vi "SW_Fire_TTL_on_start_or_stop.vi"(7 "TTL pulse length, ms":dbl=250.0 format="%#_13g", 8 "error in (no error)":errorcluster, 9 "Serial Port In":refnum<visa-resource-name>="COM3", 10 "Flush receive buffer?":bool=TRUE, 11 "IO parameters cluster in":T1) -> (0 "error out":errorcluster, 1 "Serial Port Out":refnum<visa-resource-name>="COM3", 3 "Time spent to process command, s":dbl=250.0)   [LabVIEW 2018, in "Tracker.lvlib"]
doc: "Fires TTL High to the TTL2 output for ~250 ms (default)."
uses:
  Tracker.lvlib
  Controls/CTL_IO_params_cluster.ctl
  <vilib>/Instr/_visa.llb/VISA Flush IO Buffer Mask.ctl
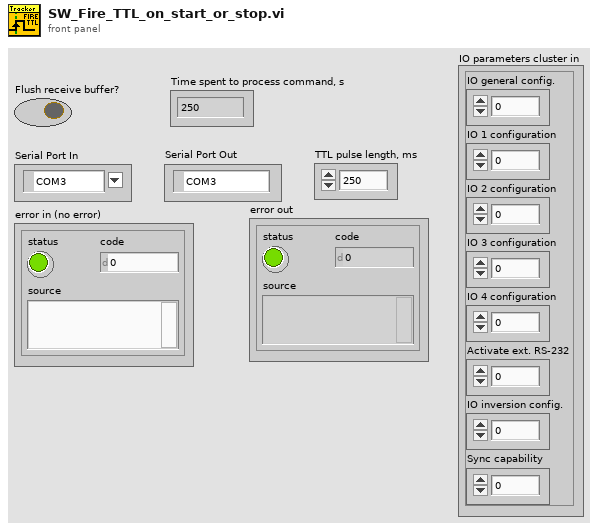
[diagram p1: front panel]
types:
  T1 = typedef "Tracker.lvlib/CTL_IO_params_cluster.ctl" = cluster{"IO general config.":u16, "IO 1 configuration":u16, "IO 2 configuration":u16, "IO 3 configuration":u16, "IO 4 configuration":u16, "Activate ext. RS-232":u16, "IO inversion config.":u16, "Sync capability":u8}
  T2 = typedef "VISA Flush IO Buffer Mask.ctl" = u16
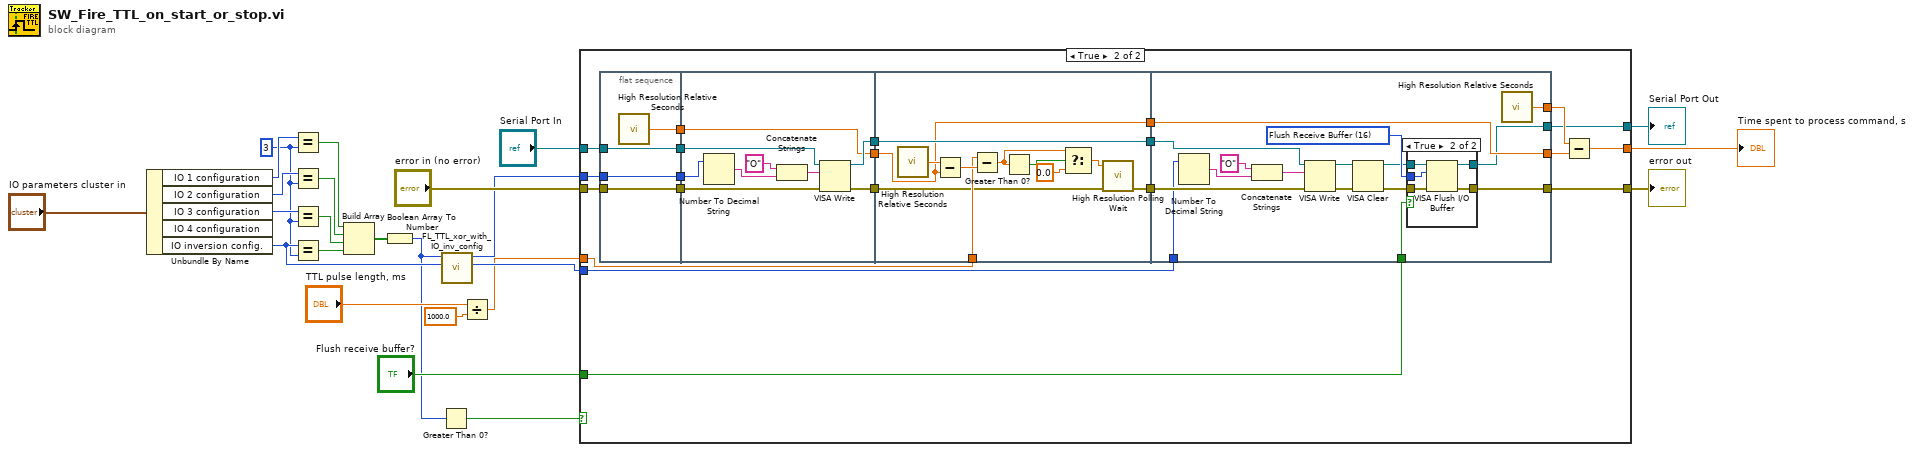
[diagram p0: block diagram]
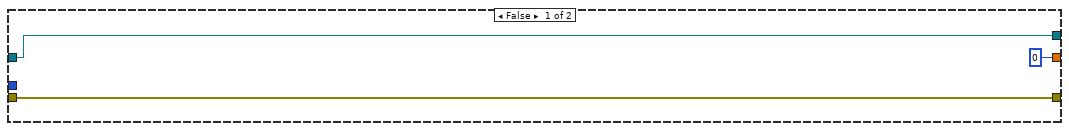
[diagram p2: hidden frame]
diagram:
  w12 = u16 3
  n1 = Unbundle By Name("IO parameters cluster in") -> ("IO 1 configuration"=w16:u16, "IO 2 configuration"=w15:u16, "IO 3 configuration"=w14:u16, "IO inversion config."=w13:u16)  [unwired: 1 out]
  n2 = Equal?(x=w16, y=w12) -> (x = y?=w11:bool)
  n3 = Equal?(x=w15, y=w12) -> (x = y?=w10:bool)
  n4 = Equal?(x=w14, y=w12) -> (x = y?=w9:bool)
  n5 = Equal?(x=w13, y=w12) -> (x = y?=w8:bool)
  n6 = Build Array(w11, w10, w9, w8) -> (w7:bool[])
  n7 = Boolean Array To Number(Boolean array=w7) -> (number=w6:u32)
  n8 = Greater Than 0?(x=w6) -> (x > 0?=w5:bool)
  n9 = call "FL_TTL_xor_with_IO_inv_config.vi"("IO inversion config."=w13, "TTL port(s) config to fire"=w6) -> ("OFF config."=w3:u32, "ON config."=w4:u32)  [unwired: 8 in]
  n10 = Divide(x="TTL pulse length, ms", y=1000.0) -> (x/y=w2:dbl)
  n11 = case shown="True" w5 {
    tunnel: [u32 0 w40] -> w24
    tunnel: [w26 w39] -> w23
    tunnel: "Serial Port In" -> [w26 w38]
    tunnel: "Flush receive buffer?" -> [_ w37]
    tunnel: [w25 w36] -> w20
    tunnel: "error in (no error)" -> [w25 w35]
    tunnel: w4 -> [_ w34]
    tunnel: w2 -> [_ w33]
    tunnel: w3 -> [_ w32]
    frame False {
    }
    frame True {
      n12 = flat-sequence {
        tunnel: w34 -> [w50]
        tunnel: w35 -> [w51]
        tunnel: w38 -> [w52]
        tunnel: [w52] -> w31
        tunnel: [w49] -> w30
        tunnel: [w51] -> w29
        tunnel: [w50] -> w28
        tunnel: [w61] -> w48
        tunnel: [w60] -> w47
        tunnel: [w58] -> w44
        tunnel: w31 -> [w59]
        tunnel: w30 -> [w58]
        tunnel: w29 -> [w57]
        tunnel: w28 -> [w54]
        tunnel: [w72] -> w46
        tunnel: w48 -> [w72]
        tunnel: [w63] -> w45
        tunnel: w47 -> [w64]
        tunnel: w44 -> [w66]
        tunnel: [w66] -> w41
        tunnel: w33 -> [w65]
        tunnel: [w79] -> w36
        tunnel: [w78] -> w39
        tunnel: [w87] -> w42
        tunnel: [w88] -> w43
        tunnel: w37 -> [w86]
        tunnel: w41 -> [w87]
        tunnel: w45 -> [w85]
        tunnel: w46 -> [w84]
        tunnel: w32 -> [w73]
        frame #0 {
          n13 = call <vilib>:"High Resolution Relative Seconds.vi"() -> ("relative seconds"=w49:dbl)
        }
        frame #1 {
          n14 = Number To Decimal String(number=w54) -> (decimal integer string=w56:string)  [unwired: 1 in]
          n15 = Concatenate Strings("O" ("string"), w56) -> (w53:string)
          n16 = VISA Write(VISA resource name=w59, write buffer=w53, error in (no error)=w57) -> (VISA resource name out=w61:refnum<visa-resource-name>, error out=w60:errorcluster)  [unwired: 1 out]
        }
        frame #2 {
          n17 = call <vilib>:"High Resolution Relative Seconds.vi"() -> ("relative seconds"=w71:dbl)
          n18 = Subtract(x=w71, y=w66) -> (x-y=w70:dbl)
          n19 = Subtract(x=w65, y=w70) -> (x-y=w68:dbl)
          n20 = Greater Than 0?(x=w68) -> (x > 0?=w69:bool)
          n21 = Select(t=w68, s=w69, f=0.0) -> (s? t:f=w62:dbl)
          n22 = call <vilib>:"High Resolution Polling Wait.vi"("error in (no error)"=w64, "seconds to wait"=w62) -> ("error out"=w63:errorcluster)  [unwired: 9 in]
        }
        frame #3 {
          w81 = T2 16 items=["Flush Receive Buffer"=16, "Write Transmit Buffer to Device"=32, "Flush Receive Buffer (No I/O)"=64, "Flush Transmit Buffer"=128] ("Mask")
          n23 = Number To Decimal String(number=w73) -> (decimal integer string=w76:string)  [unwired: 1 in]
          n24 = Concatenate Strings("O" ("string"), w76) -> (w74:string)
          n25 = VISA Write(VISA resource name=w84, write buffer=w74, error in (no error)=w85) -> (VISA resource name out=w83:refnum<visa-resource-name>, error out=w82:errorcluster)  [unwired: 1 out]
          n26 = VISA Clear(VISA resource name=w83, error in (no error)=w82) -> (VISA resource name out=w80:refnum<visa-resource-name>, error out=w77:errorcluster)
          n27 = case shown="True" w86 {
            tunnel: [w90 w92] -> w78
            tunnel: [w89 w93] -> w79
            tunnel: w81 -> [_ w95]
            tunnel: w80 -> [w90 w94]
            tunnel: w77 -> [w89 w91]
            frame False {
            }
            frame True {
              n28 = VISA Flush I/O Buffer(VISA resource name=w94, mask (16)=w95, error in (no error)=w91) -> (VISA resource name out=w92:refnum<visa-resource-name>, error out=w93:errorcluster)
            }
          }
          n29 = call <vilib>:"High Resolution Relative Seconds.vi"() -> ("relative seconds"=w88:dbl)
        }
      }
      n30 = Subtract(x=w43, y=w42) -> (x-y=w40:dbl)
    }
  }
  "Time spent to process command, s" <- w24
  "Serial Port Out" <- w23
  "error out" <- w20
